vi "signaling node test.vi"() -> ()   [LabVIEW 2019]
panel:
  out "loop 1 iterations":i32
  out "loop 2 iterations":i32
  in  "Numeric":i32=10
  in  "Boolean":bool
  in  "stop":bool
  out "x+1":dbl
  in  "Test":bool
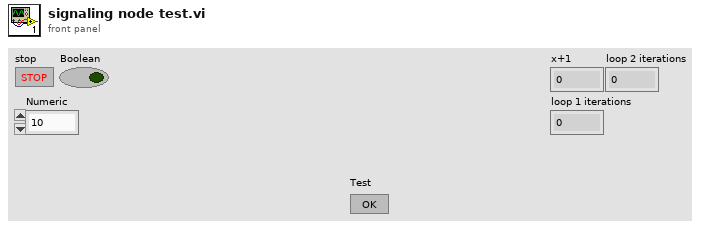
[diagram p1: front panel]
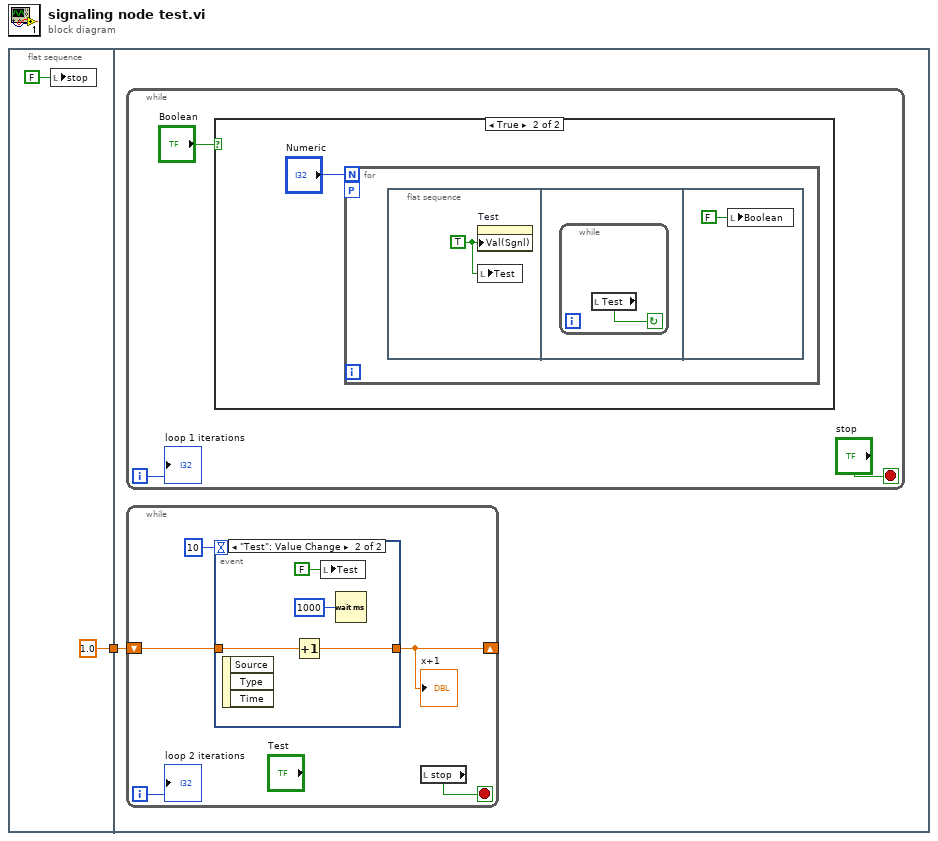
[diagram p0: block diagram]
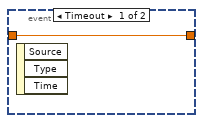
[diagram p2: hidden frame]
diagram:
  n1 = flat-sequence {
    tunnel: [1.0] -> w1
    tunnel: w1 -> [w4]
    frame #0 {
      n2 = local write "stop"(FALSE ("stop")) -> ()
    }
    frame #1 {
      n3 = while {
        i -> [w15]
        stop <- "stop" stop-if-true
        n4 = case shown="True" "Boolean" {
          frame False {
          }
          frame True {
            n5 = for {
              N: "Numeric" -> [_]
              workers-P: _ -> [_]
              n6 = flat-sequence {
                frame #0 {
                  w19 = TRUE ("Test")
                  n7 = property on="Test" class="Bool (strict)"("Val(Sgnl)"=w19) -> ()  [unwired: 2 in, 2 out]
                  n8 = local write "Test"(w19) -> ()
                }
                frame #1 {
                  n9 = while {
                    stop <- w20 continue-if-true
                    n10 = local read "Test"() -> (w20:bool)
                  }
                }
                frame #2 {
                  n11 = local write "Boolean"(FALSE ("Test")) -> ()
                }
              }
            }
          }
        }
        "loop 1 iterations" <- w15
      }
      n12 = while {
        shift-right: [w8] -> _
        shift-left: w4 -> [w9]
        i -> [w5]
        stop <- w7 stop-if-true
        n13 = event shown="[1] \"Test\": Value Change" {
          selector: _ -> [_ _]
          dyn-events: _ -> [_ _]
          timeout: 10 -> [_ _]
          tunnel: w9 -> [w10 w14]
          tunnel: [w10 w13] -> w8
          event Timeout {
            n14 = event-data() -> ()  [unwired: 1 in, 3 out]
          }
          event "Test": Value Change {
            n15 = event-data() -> ()  [unwired: 1 in, 3 out]
            n16 = Increment(x=w14) -> (x+1=w13:dbl)
            n17 = local write "Test"(FALSE ("Test")) -> ()
            n18 = Wait (ms)(milliseconds to wait=u32 1000) -> ()  [unwired: 1 out]
          }
        }
        "x+1" <- w8
        n19 = local read "stop"() -> (w7:bool)
        "loop 2 iterations" <- w5
      }
    }
  }
